vi "Defer Panel Updates.vi"(8 "error in (no error)":errorcluster, 11 "IViewManager In":refnum<class "IViewManager.lvclass">) -> (0 "error out":errorcluster, 3 "IViewManager Out":refnum<class "IViewManager.lvclass">)   [LabVIEW 2015, in "IViewManager.lvlib" / "IViewManager.lvclass"]
uses:
  IViewManager.lvclass
  IViewManager.lvclass/IViewManager.ctl
  <vilib>/ActorFramework/Message Enqueuer/Message Enqueuer.lvclass/Message Enqueuer.ctl
  <vilib>/ActorFramework/Message Enqueuer/Enqueue.vi
  <vilib>/ActorFramework/Message Priority Queue/Priority Enqueue.vi
  IViewable/IViewable/IViewable.lvclass
  IViewable/IViewable Messages/Defer Panel Updates Msg/Defer Panel Updates Msg.lvclass
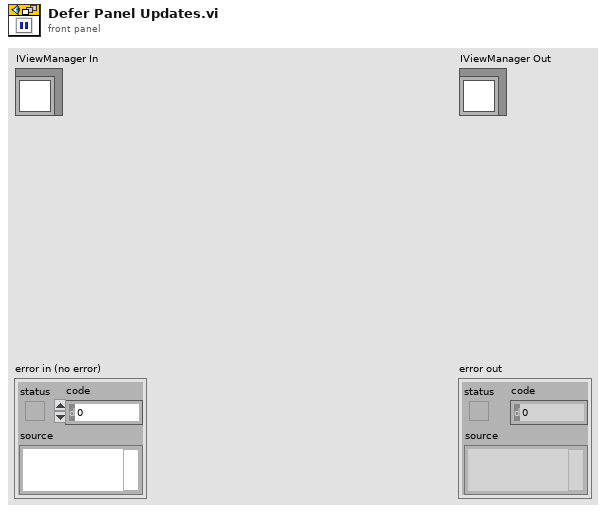
[diagram p1: front panel]
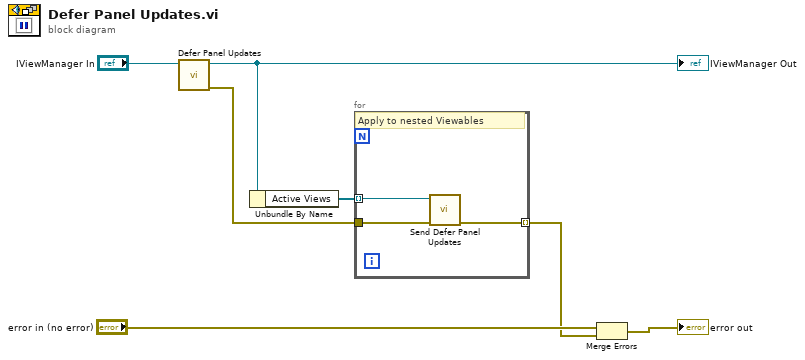
[diagram p0: block diagram]
diagram:
  n1 = call-parent "Defer Panel Updates.vi"("IViewable In"="IViewManager In") -> ("error out"=w2:errorcluster, "IViewable Out"=w6:refnum<class "IViewManager.lvclass">)  [unwired: 9 in]
  "IViewManager Out" <- w6
  n2 = Unbundle By Name(w6) -> ("Active Views"=w5:refnum<class "Message Enqueuer.lvclass">[])
  n3 = for {
    tunnel: w5 -> [w8] mode=indexing
    tunnel: w2 -> [w10]
    tunnel: [w9] -> w1 mode=indexing
    # "Apply to nested Viewables"
    n4 = call "Send Defer Panel Updates.vi"("error in (no error)"=w10, "Message Enqueuer"=w8) -> ("error out"=w9:errorcluster)  [unwired: 8 in, 1 out]
  }
  n5 = Merge Errors("error in (no error)", w1) -> (→"error out":errorcluster)
